vi "LOG txt.vi"(8 "error in (no error)":errorcluster, 10 "Leds 2":bool[](array[boolean]), 11 "Login bin in":refnum<class "Login bin.lvclass">) -> (0 "error out":errorcluster, 3 "Login bin out":refnum<class "Login bin.lvclass">)   [LabVIEW 2020, in "Login bin.lvlib" / "Login bin.lvclass"]
uses:
  Login bin.lvclass
  Login bin.lvclass/Login bin.ctl
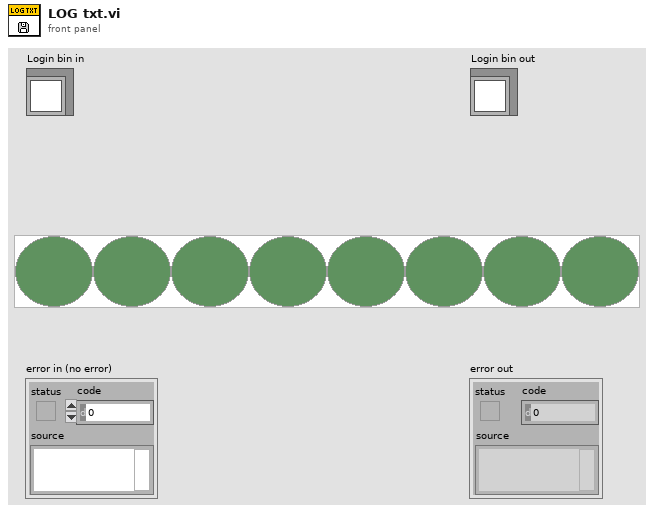
[diagram p1: front panel]
types:
  T1 = enum16{"open", "replace", "create", "open or create", "replace or create", "replace or create with confirmation"}
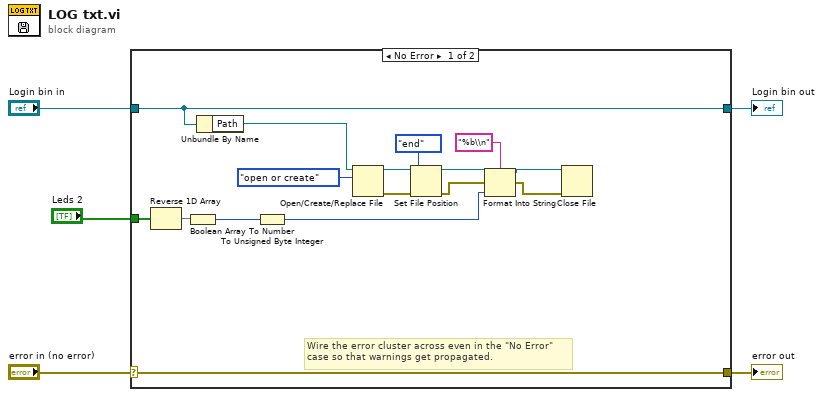
[diagram p0: block diagram]
diagram:
  n1 = case shown="No Error" "error in (no error)" {
    selector: "error in (no error)" -> [w21 w23]
    tunnel: [w21 w23] -> w4
    tunnel: [w20 w22] -> w2
    tunnel: "Login bin in" -> [w20 w22]
    tunnel: "Leds 2" -> [w7 _]
    frame No Error {
      # "Wire the error cluster across even in the \"No Error\"\ncase so that warnings get propagated."
      n2 = Reverse 1D Array(array=w7) -> (reversed array=w6:bool[])
      n3 = Boolean Array To Number(Boolean array=w6) -> (number=w9:u32)
      n4 = Unbundle By Name(w20) -> ("Path"=w11:path)
      n5 = To Unsigned Byte Integer(number=w9) -> (unsigned 8bit integer=w8:u8)
      n6 = Open/Create/Replace File(file path (use dialog)=w11, operation (0:open)=T1."open or create") -> (refnum out=w15:refnum<file>, error out=w16:errorcluster)  [unwired: 4 in, 1 out]
      n7 = Set File Position(refnum=w15, from (0:start)=enum16{"start", "end", "current"}."end", error in=w16) -> (refnum out=w14:refnum<file>, error out=w13:errorcluster)  [unwired: 1 in]
      n8 = Format Into String(format string="%b\\n", initial string=w14, error in=w13, w8) -> (resulting string=w18:refnum<file>, error out=w17:errorcluster)
      n9 = Close File(refnum=w18, error in=w17) -> ()  [unwired: 2 out]
    }
    frame Error {
    }
  }
  "error out" <- w4
  "Login bin out" <- w2
